vi "ExPickStripADC.vi"() -> ()   [LabVIEW 2010]
panel:
  in  "Readout Port":i32=-1 min=-1 step=1
  in  "ADC Offset":i32=-1 min=-1 step=1
  in  "ADC Gain":i32=-1 min=-1 step=1
  in  "ADC speed":i32=-2 min=-3 step=1
  in  "Trigger Edge":u32(ring)=1 items=["", "Positive (leading) edge", "Negative (falling) Edge"]
  in  "Trigger/Timing Mode":u32(ring)=1 items=["N/A", "FreeRun/Timed", "Single Trigger (PM only)", "Ext Sync/Strobed", "Bulb (PM only)", "Variable (PM only)", "Flash Mode (PM only)"]
  in  "Strip":u32=1 min=1 step=1
  out "Strip":sgl[](graph)
  in  "Temperature":dbl=-10.0 format="%.2f"
  in  "Exposure":dbl min=0.0 step=0.001 format="%.3f"
  in  "stop":bool
  out "error out":errorcluster
  in  "error in (no error)":errorcluster
  # "ExPickStrip:\nThis example allows a strip to be picked before running. \nIt will then program up the strip and display it on the graph.\nNote: This example uses circular buffers, so camera must\nsupport circular buffers."
  # "For Slowest ADC speed set this to -3\nFor Fastest ADC speed set this to -2\nTo use current ADC speed don't  hook up or use -1\notherwise put speed in as kHz"
  # "To use current gain don't hook up or set to -1"
  # "To use current gain don't hook up or set to -1"
  # "To use current gain don't hook up or set to -1"
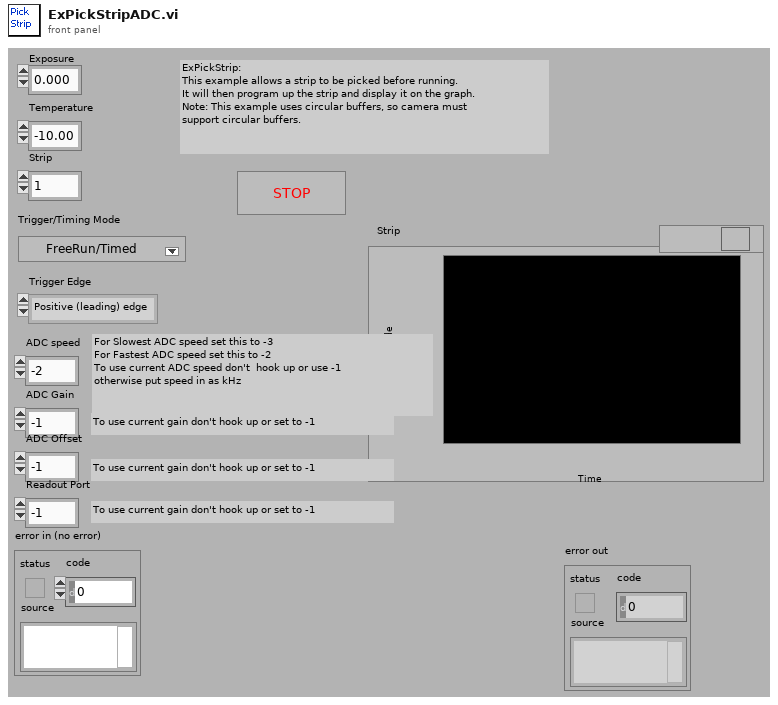
[diagram p1: front panel]
types:
  T1 = cluster{"Acquire Mode \n(1-Focus sync)\nNote: not all \ncamera support \nthis mode.":i32, "Exposure":dbl, "Number of frames":i32, "Software Accumulations":i32}
  T2 = cluster{"Camera Handle":u32, "Pulser Handle":u32, "File Handle":u32, "Display Handle":u32, "Image Handle":u32}
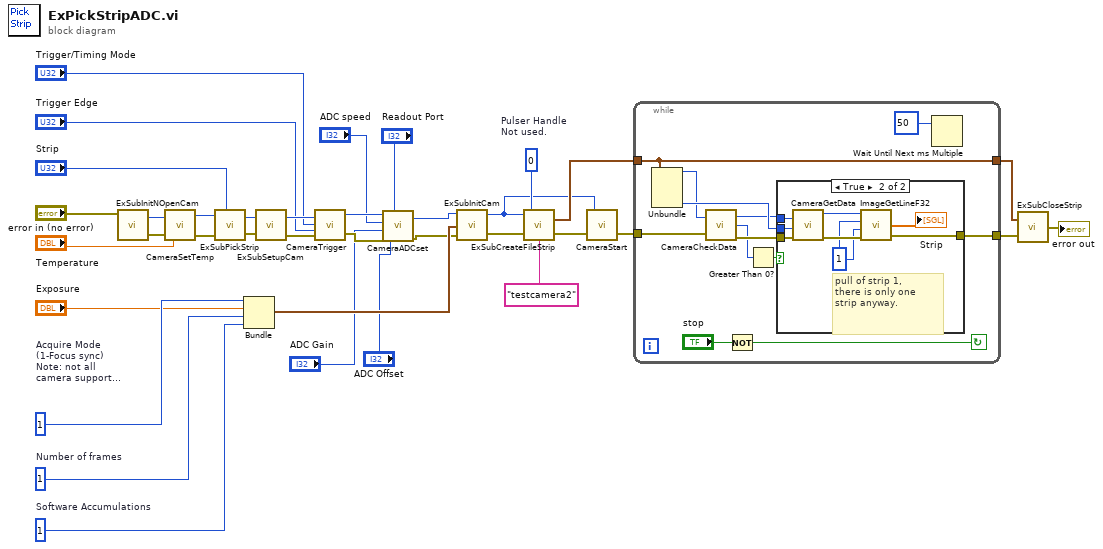
[diagram p0: block diagram]
diagram:
  w28 = 0  # Pulser Handle Not used.
  w34 = 1  # Number of frames
  w35 = 1  # Acquire Mode  (1-Focus sync) Note: not all  camera support  this mode.
  w33 = 1  # Software Accumulations
  n1 = call "ExSubInitNOpenCam.vi"("error in (no error)"="error in (no error)") -> ("Camera Handle"=w16:u32, "error out"=w17:errorcluster)
  n2 = call <userlib>:"CameraSetTemp.vi"("error in (no error)"=w17, "Temperature"="Temperature", "Camera Handle"=w16) -> ("error out"=w15:errorcluster, "Camera Handle"=w14:u32)
  n3 = call "ExSubPickStrip.vi"("error in (no error)"=w15, "Strip to display"="Strip", "Camera Handle"=w14) -> ("error out"=w12:errorcluster, "Camera Handle"=w11:u32)
  n4 = Bundle("Acquire Mode \n(1-Focus sync)\nNote: not all \ncamera support \nthis mode."=w35, "Exposure"="Exposure", "Number of frames"=w34, "Software Accumulations"=w33) -> (w30:T1)  [unwired: 1 in]
  n5 = call "ExSubSetupCam.vi"("error in (no error)"=w12, "Camera Handle"=w11) -> ("error out"=w21:errorcluster, "Camera Handle"=w22:u32)
  n6 = call <userlib>:"CameraTrigger.vi"("error in"=w21, "Trigger Edge"="Trigger Edge", "Timing Mode"="Trigger/Timing Mode", "Camera Handle"=w22) -> ("error out"=w8:errorcluster, "Camera Handle"=w6:u32)
  n7 = call <userlib>:"CameraADCset.vi"("ADC offset"="ADC Offset", "Read Out port"="Readout Port", "error in (no error)"=w8, "ADC Gain"="ADC Gain", "ADC Speed"="ADC speed", "Camera Handle"=w6) -> ("error out"=w7:errorcluster, "Camera Handle"=w5:u32)
  n8 = call "ExSubInitCam.vi"("error in (no error)"=w7, "Camera Information"=w30, "Camera Handle"=w5) -> ("error out"=w29:errorcluster, "Camera Handle"=w26:u32)
  n9 = call "ExSubCreateFileStrip.vi"("error in (no error)"=w29, "File and Display Name"="testcamera2", "Pulser Handle"=w28, "Camera Handle"=w26) -> ("error out"=w19:errorcluster, "Handles Out"=w27:T2)
  n10 = call <userlib>:"CameraStart.vi"("error in"=w19, "Camera Handle"=w26) -> ("error out"=w20:errorcluster)  [unwired: 1 out]
  n11 = while {
    tunnel: w27 -> [w45]
    tunnel: w20 -> [w44]
    tunnel: [w42] -> w24
    tunnel: [w45] -> w25
    stop <- w46 continue-if-true
    n12 = Unbundle(w45) -> ("Camera Handle"=w40:u32, "Image Handle"=w41:u32)  [unwired: 3 out]
    n13 = call <userlib>:"CameraCheckData.vi"("Camera Handle"=w40, "error in"=w44) -> ("Camera Handle"=w39:u32, "Number Of Frames Available"=w37:i32, "error out"=w43:errorcluster)
    n14 = Not(x="stop") -> (.not. x?=w46:bool)
    n15 = Greater Than 0?(x=w37) -> (x > 0?=w38:bool)
    n16 = case shown="True" w38 {
      tunnel: w43 -> [w49 w56]
      tunnel: [w49 w54] -> w42
      tunnel: w41 -> [_ w51]
      tunnel: w39 -> [_ w50]
      frame False {
      }
      frame True {
        w52 = 1
        # "pull of strip 1,\nthere is only one\nstrip anyway."
        n17 = call <userlib>:"CameraGetData.vi"("error in"=w56, "Data Handle"=w51, "Camera Handle"=w50) -> ("error out"=w55:errorcluster, "Data Handle"=w53:u32)  [unwired: 1 out]
        n18 = call <userlib>:"ImageGetLineF32.vi"("error in"=w55, "Z Position"=w52, "Y Position"=w52, "Data Handle"=w53) -> ("error out"=w54:errorcluster, "Array F32"=→"Strip":sgl[])  [unwired: 1 out]
      }
    }
    n19 = Wait Until Next ms Multiple(millisecond multiple=50) -> ()  [unwired: 1 out]
  }
  n20 = call "ExSubCloseStrip.vi"("error in (no error)"=w24, "Handles In"=w25) -> ("error out"=→"error out":errorcluster)
